vi "Configure Reference.vi"(6 "External Reference Frequency (10 MHz)":dbl=10000000.0, 8 "error in (no error)":errorcluster, 9 "Reference Source (0: Internal)":u16(ring) items=["Internal", "External"], 10 "Modulation Format (1: Dual Modulation)":u16(ring)=1 items=["Dual Modulation"=1, "Dual ARB"=2, "Multitone"=3, "Two-tone"=6, "AWGN ARB"=8], 11 "VISA resource name":refnum<visa-resource-name>) -> (0 "error out":errorcluster, 3 "VISA resource name out":refnum<visa-resource-name>)   [LabVIEW 2012, in "Agilent PSG MXG Series.lvlib"]
doc: "Configures reference source and level for the specific modulation format.\n\n<B>Notes:</B>\n(1) This VI is valid only in E8267C, E8257D, E8267D, N5162A, N5182A.\n\n(2) For E8267C, this VI is valid only when the instrument installs <B>Option 002</B> (Internal baseband generator) or <B>Option 602</B> (Digital bus baseband generator).\n\n(3) For E8267D, this VI is valid only when the instrument installs <B>Option 601</B> or <B>Option 602</B> (Internal baseband generator).\n\n(4) For N5162A and N5182A, this VI is valid only when the instrument installs <B>Option 651</B> or <B>Option 652</B> or <B>Option 654</B> (Internal baseband generator)."
uses:
  <instrlib>/Agilent PSG MXG Series/Agilent PSG MXG Series.lvlib
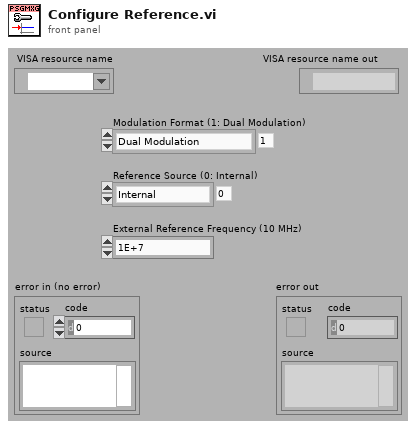
[diagram p1: front panel]
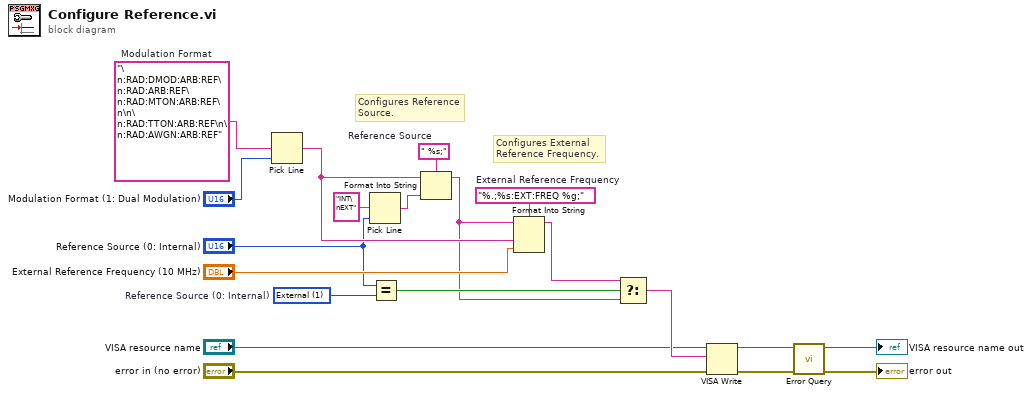
[diagram p0: block diagram]
diagram:
  w11 = u16 1 items=["Internal", "External"]  # Reference Source (0: Internal)
  w15 = "%.;%s:EXT:FREQ %g;"  # External Reference Frequency
  w18 = " %s;"  # Reference Source
  w20 = "\n:RAD:DMOD:ARB:REF\n:RAD:ARB:REF\n:RAD:MTON:ARB:REF\n\n\n:RAD:TTON:ARB:REF\n\n:RAD:AWGN:ARB:REF"  # Modulation Format
  # "Configures External\nReference Frequency."
  # "Configures Reference\nSource."
  n1 = Pick Line(multi-line string=w20, line index="Modulation Format (1: Dual Modulation)") -> (output string=w14:string)  [unwired: 1 out]
  n2 = Pick Line(multi-line string="INT\nEXT", line index="Reference Source (0: Internal)") -> (output string=w17:string)  [unwired: 1 out]
  n3 = Equal?(x="Reference Source (0: Internal)", y=w11) -> (x = y?=w10:bool)
  n4 = Format Into String(format string=w18, initial string=w14, w17) -> (resulting string=w8:string)  [unwired: 1 in, 1 out]
  n5 = Format Into String(format string=w15, initial string=w8, w14, "External Reference Frequency (10 MHz)") -> (resulting string=w9:string)  [unwired: 1 in, 1 out]
  n6 = Select(t=w9, s=w10, f=w8) -> (s? t:f=w7:string)
  n7 = VISA Write(VISA resource name="VISA resource name", write buffer=w7, error in (no error)="error in (no error)") -> (VISA resource name out=w6:refnum<visa-resource-name>, error out=w5:errorcluster)  [unwired: 1 out]
  n8 = call <instrlib>:"Error Query.vi"("error in (no error)"=w5, "VISA resource name"=w6) -> ("error out"=→"error out":errorcluster, "VISA resource name out"=→"VISA resource name out":refnum<visa-resource-name>)  [unwired: 8 out]
